vi "t_settle RC.vi"(10 "filter order":i32, 11 "time constant (s)":dbl) -> (3 "f -3 dB (Hz)":dbl)   [LabVIEW 2019, in "DSP.lvclass"]
uses:
  DSP.lvclass
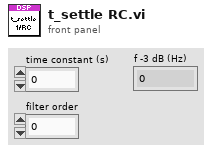
[diagram p1: front panel]
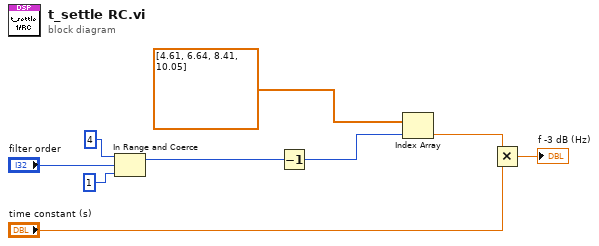
[diagram p0: block diagram]
diagram:
  n1 = In Range and Coerce(upper limit=4 ("lower limit"), x="filter order", lower limit=1) -> (coerced(x)=w6:i32)  [unwired: 1 out]
  n2 = Decrement(x=w6) -> (x-1=w5:i32)
  n3 = Index Array(array=dbl[] [4.61, 6.64, 8.41, 10.05], index=w5) -> (element=w2:dbl)
  n4 = Multiply(x=w2, y="time constant (s)") -> (x*y=→"f -3 dB (Hz)":dbl)
